vi "SetPNGimage.vi"(8 "Error out":errorcluster, 9 "Glyph Index":i32=1, 10 "path to PNG file":path, 11 "Tree in":refnum<class "Tree.lvclass">) -> (0 "Error out":errorcluster, 3 "Tree out":refnum<class "Tree.lvclass">)   [LabVIEW 2021, in "Tree.lvlib" / "Tree.lvclass"]
uses:
  Tree.lvclass
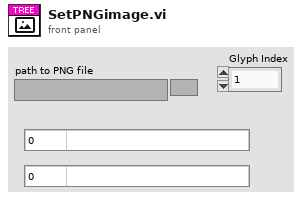
[diagram p1: front panel]
types:
  T1 = typedef "imagedata.ctl" = cluster{"image type":i32, "image depth":i32, "image":u8[], "mask":u8[], "colors":u32[], "Rectangle":cluster{"left":i16, "top":i16, "right":i16, "bottom":i16}}
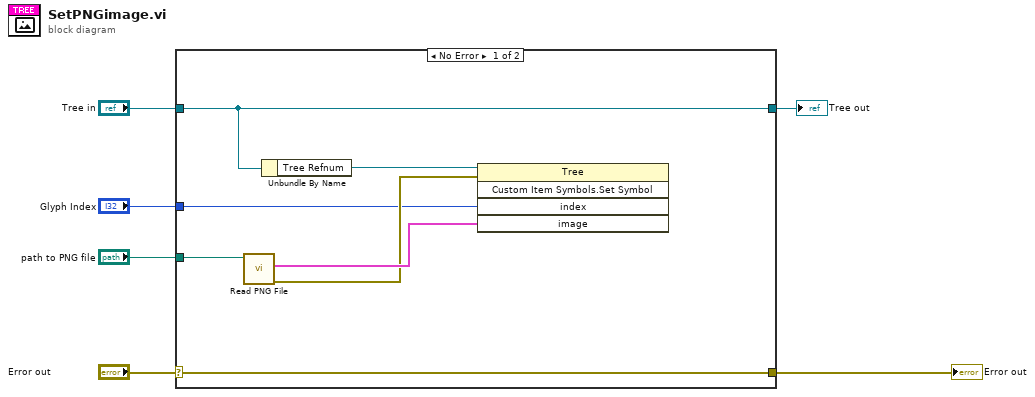
[diagram p0: block diagram]
diagram:
  n1 = case shown="No Error" "Error out" {
    selector: "Error out" -> [w13 w15]
    tunnel: [w13 w15] -> w5
    tunnel: [w12 w14] -> w3
    tunnel: "Tree in" -> [w12 w14]
    tunnel: "path to PNG file" -> [w10 _]
    tunnel: "Glyph Index" -> [w7 _]
    frame No Error {
      n2 = call <vilib>:"Read PNG File.vi"("path to PNG file"=w10) -> ("error out"=w8:errorcluster, "image data"=w9:T1)  [unwired: 8 in, 1 out]
      n3 = Unbundle By Name(w12) -> ("Tree Refnum"=w11:refnum<vi>)
      n4 = invoke on="Invoke Node" class="Tree" method="Custom Item Symbols.Set Symbol"(reference=w11, error in=w8, "index"=w7, "image"=w9) -> ()  [unwired: 1 in, 5 out]
    }
    frame Error {
    }
  }
  "Error out" <- w5
  "Tree out" <- w3
